vi "get_dimensions.vi"(8 "error in (no error)":errorcluster, 11 "PointCollection in":refnum<class "PointCollection.lvclass">) -> (0 "error out":errorcluster, 1 "y":dbl[](array[numeric]), 2 "x":dbl[](array[numeric]), 3 "PointCollection out":refnum<class "PointCollection.lvclass">, 4 "z":dbl[](array[numeric]), 6 "IDs":dbl[](array[numeric]))   [LabVIEW 2010, in "PointCollection.lvclass"]
uses:
  PointCollection.lvclass
  mode_enum.ctl
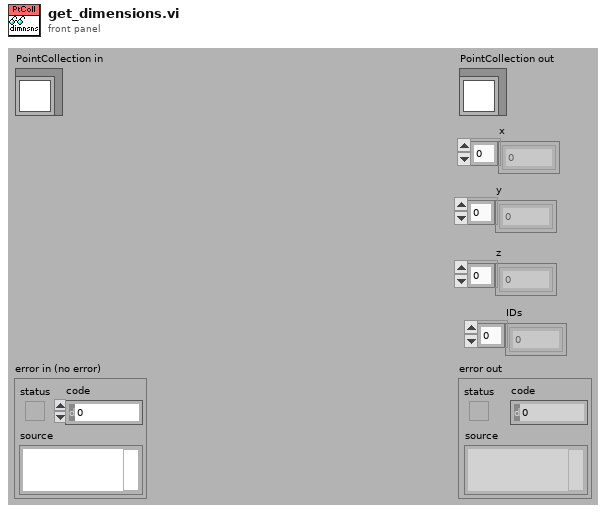
[diagram p1: front panel]
types:
  T1 = typedef "PointCollection.lvclass/mode_enum.ctl" = enum16{"points first", "dimensions first"}
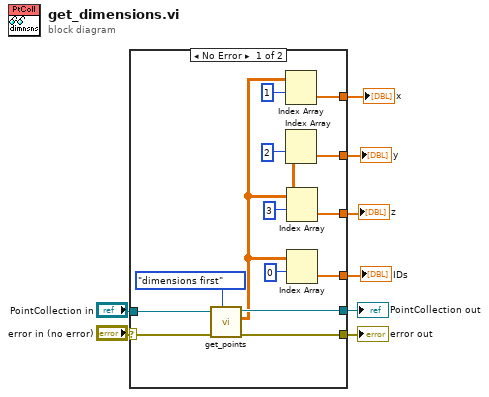
[diagram p0: block diagram]
diagram:
  n1 = case shown="No Error" "error in (no error)" {
    selector: "error in (no error)" -> [w22 w24]
    tunnel: [w19 w24] -> w7
    tunnel: [w20 w23] -> w5
    tunnel: "PointCollection in" -> [w21 w23]
    tunnel: [w18 _] -> w4
    tunnel: [w17 _] -> w3
    tunnel: [w16 _] -> w2
    tunnel: [w15 _] -> w1
    frame No Error {
      n2 = call-dynamic "get_points.vi"("retrieval mode"=mode_enum."dimensions first", "error in (no error)"=w22, "PointCollection in"=w21) -> ("error out"=w19:errorcluster, "points"=w10:dbl[][], "PointCollection out"=w20:refnum<class "PointCollection.lvclass">)  [unwired: 6 in]
      n3 = Index Array(array=w10, index (row)=1) -> (element=w18:dbl[])  [unwired: 1 in]
      n4 = Index Array(array=w10, index (row)=2) -> (element=w17:dbl[])  [unwired: 1 in]
      n5 = Index Array(array=w10, index (row)=3) -> (element=w16:dbl[])  [unwired: 1 in]
      n6 = Index Array(array=w10, index (row)=0) -> (element=w15:dbl[])  [unwired: 1 in]
    }
    frame Error {
    }
  }
  "error out" <- w7
  "PointCollection out" <- w5
  "x" <- w4
  "y" <- w3
  "z" <- w2
  "IDs" <- w1
